vi "Debug_Convert_Data_to_String.vi"(8 "error in (no error)":errorcluster, 11 "AB_Source_Library in":refnum<class "AB_Source_Library.lvclass">) -> (0 "error out":errorcluster, 1 "classData":string, 2 "sourceType":string, 3 "AB_Source_Library out":refnum<class "AB_Source_Library.lvclass">)   [LabVIEW 2020, in "AB_Source_Library.lvclass"]
uses:
  <vilib>/AppBuilder/AB_Classes/Source/Library/AB_Source_Library.lvclass
  <vilib>/AppBuilder/AB_Classes/Source/Library/AB_Source_Library.lvclass/AB_Source_Library.ctl
  <vilib>/AppBuilder/AB_Classes/Source/AB_Source.lvclass
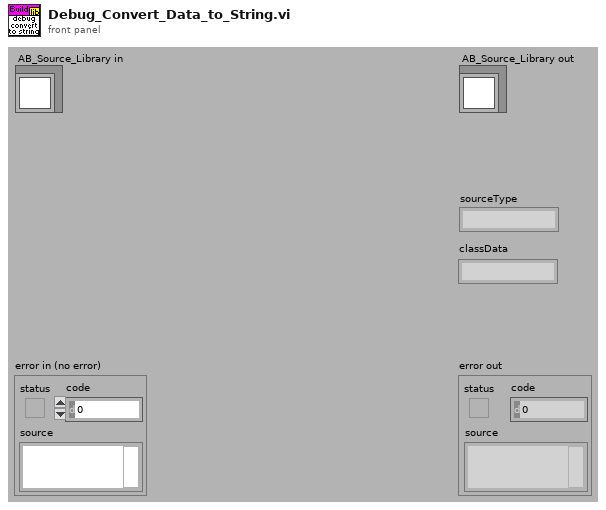
[diagram p1: front panel]
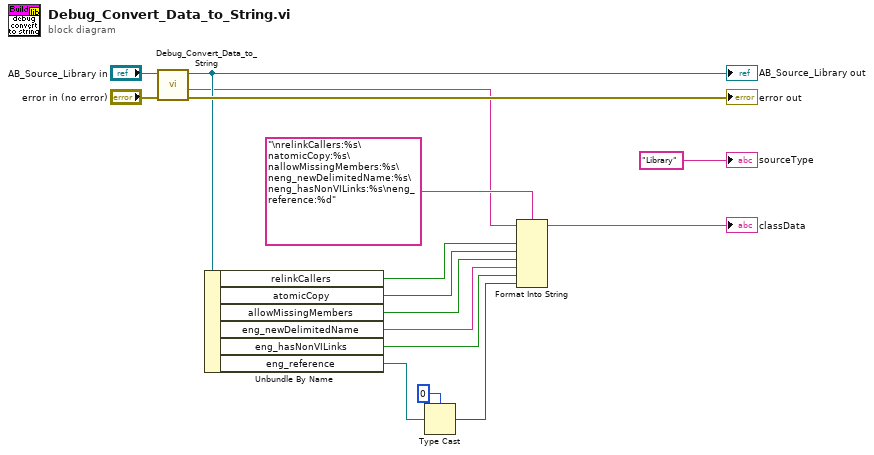
[diagram p0: block diagram]
diagram:
  n1 = call-parent "Debug_Convert_Data_to_String.vi"("error in (no error)"="error in (no error)", "AB_Source in"="AB_Source_Library in") -> ("error out"=→"error out":errorcluster, "classData"=w2:string, "AB_Source out"=w5:refnum<class "AB_Source_Library.lvclass">)  [unwired: 6 in, 1 out]
  "AB_Source_Library out" <- w5
  n2 = Unbundle By Name(w5) -> ("relinkCallers"=w12:bool, "atomicCopy"=w11:bool, "allowMissingMembers"=w1:bool, "eng_newDelimitedName"=w10:string, "eng_hasNonVILinks"=w9:bool, "eng_reference"=w8:refnum<vi>)
  n3 = Type Cast(type=u32 0, x=w8) -> (*(type *) &x=w6:u32)
  n4 = Format Into String(format string="\nrelinkCallers:%s\natomicCopy:%s\nallowMissingMembers:%s\neng_newDelimitedName:%s\neng_hasNonVILinks:%s\neng_reference:%d", initial string=w2, w12, w11, w1, w10, w9, w6) -> (resulting string=→"classData":string)  [unwired: 1 in, 1 out]
  "sourceType" <- "Library"
